vi "StringToFloat (SubVI).vi"(11 "String in":string) -> (3 "Numeric":sgl)   [LabVIEW 2017, in "LV_Unicorn.lvlib"]
uses:
  LV_Unicorn.lvlib
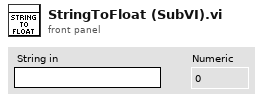
[diagram p1: front panel]
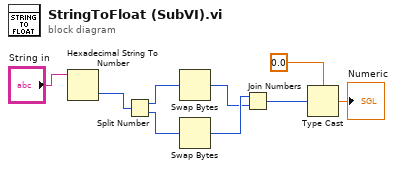
[diagram p0: block diagram]
diagram:
  n1 = Hexadecimal String To Number(string="String in") -> (number=w5:u32)  [unwired: 2 in, 1 out]
  n2 = Split Number(x=w5) -> (hi(x)=w6:u16, lo(x)=w7:u16)
  n3 = Swap Bytes(anything=w6) -> (byte swapped=w8:u16)
  n4 = Swap Bytes(anything=w7) -> (byte swapped=w9:u16)
  n5 = Join Numbers(hi=w9, lo=w8) -> ((hi.lo)=w2:u32)
  n6 = Type Cast(type=sgl 0.0, x=w2) -> (*(type *) &x=→"Numeric":sgl)
